vi "Close.vi"(8 "error in (no error)":errorcluster, 11 "TroSpec in":refnum<class "PL ISTEQ TroSpec.lvclass">) -> (0 "error out":errorcluster)   [LabVIEW 2015, in "PL ISTEQ TroSpec.lvclass"]
doc: "Closes connection to device."
uses:
  PL ISTEQ TroSpec.lvclass
  PL ISTEQ TroSpec.lvclass/PL ISTEQ TroSpec.ctl
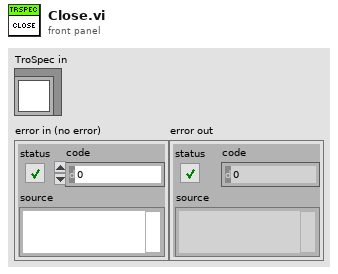
[diagram p1: front panel]
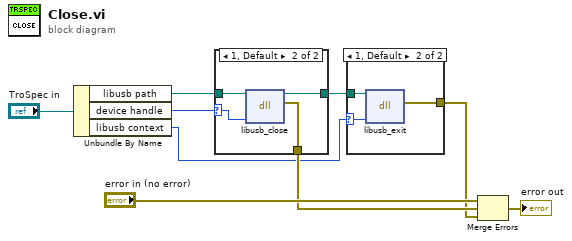
[diagram p0: block diagram]
diagram:
  n1 = Unbundle By Name("TroSpec in") -> ("libusb path"=w7:path, "device handle"=w2:u64, "libusb context"=w1:u64)
  n2 = case shown="1, Default" w2 {
    selector: w2 -> [_ w11]
    tunnel: w7 -> [w10 w14]
    tunnel: [w10 w13] -> w6
    tunnel: [_ w12] -> w4
    frame 0 {
    }
    frame 1, Default {
      n3 = dll-call lib="D:/GitHub/temp/isteq-trospec-labview/Public/libusb-1.0-x64.dll" fn="libusb_close"(path in=w14, "dev_handle"=w11) -> (path out=w13:path, error out=w12:errorcluster)  [unwired: 4 in]
    }
  }
  n4 = case shown="1, Default" w1 {
    selector: w1 -> [_ w15]
    tunnel: w6 -> [_ w17]
    tunnel: [_ w16] -> w3
    frame 0 {
    }
    frame 1, Default {
      n5 = dll-call lib="D:/GitHub/temp/isteq-trospec-labview/Public/libusb-1.0-x64.dll" fn="libusb_exit"(path in=w17, "ctx"=w15) -> (error out=w16:errorcluster)  [unwired: 4 in, 1 out]
    }
  }
  n6 = Merge Errors("error in (no error)", w4, w3) -> (→"error out":errorcluster)
